vi "EXTToU32.vi"(5 "Number":ext format="%#.6f") -> (1 "Unsigned 32-bit integer":u32, 2 "Overflow?":bool, 3 "Exact conversion?":bool)   [LabVIEW 2017, in "GPOverflow.lvlib"]
doc: "Converts <B>Number</B> to U32 keeping track of numeric overflow and exactness of conversion.\n\n<B>Exact conversion?</B> will be True only if a conversion back into the original data type of <B>Number</B> will yield the exact same number, i.e. no precision was lost during the conversion.\n\n<B>Overflow?</B> will be True if positive or negative overflow occurred. The numeric output will saturate in case of overflow.\n\nThis VI is inlined.\n\nSteen Schmidt\nGPower\n6/3 2013"
uses:
  GPOverflow.lvlib
  Comparison/GPComparison.lvlib
  Comparison/Library/IsInt/IsIntEXT.vi
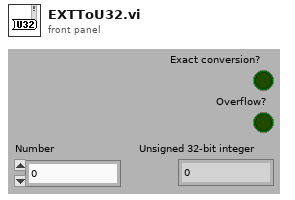
[diagram p1: front panel]
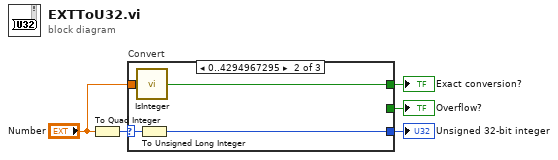
[diagram p0: block diagram]
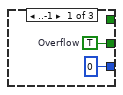
[diagram p2: hidden frame]
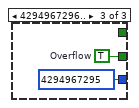
[diagram p3: hidden frame]
diagram:
  n1 = To Quad Integer(1:"Number") -> (0:w3:i64)
  n2 = case "Convert" shown="0..4294967295" w3 {
    selector: w3 -> [_ w11 _]
    tunnel: [u32 0 w10 u32 4294967295] -> w5
    tunnel: [w6 _ w12] -> w4
    tunnel: [_ w9 _] -> w2
    tunnel: "Number" -> [_ w8 _]
    frame ..-1 {
      w6 = TRUE  # Overflow
    }
    frame 0..4294967295 {
      n3 = call-poly "IsInteger.vi"("x"=w8) -> ("Integer?"=w9:bool)  [unwired: 4 in]
      n4 = To Unsigned Long Integer(number=w11) -> (unsigned 32bit integer=w10:u32)
    }
    frame 4294967296.. {
      w12 = TRUE  # Overflow
    }
  }
  "Unsigned 32-bit integer" <- w5
  "Overflow?" <- w4
  "Exact conversion?" <- w2
